vi "Final Project.vi"   [LabVIEW 2016, in "NEWNEW.lvrbt"]
uses:
  OneDrive/Documents/LabVIEW Data/NXTRobotics/Projects/NEWNEW/NEWNEW.lvrbt
  <vilib>/NXT/Block Support/NXT_InputPort.ctl
  <vilib>/NXT/Block Support/NXT_ButtonSelector.ctl
  <vilib>/NXT/Block Support/NXT_OutputPort.ctl
  <vilib>/NXT/Dual Mode Library/Sensors/EV3_Ultrasonic_CM.vi
  <vilib>/NXT/Dual Mode Library/Sensors/Light_On.vi
  <vilib>/NXT/NXTIO Xnodes/NXTIONodeSubVIs/NXTMoveMotors.vi
  <vilib>/NXT/NXTIO Xnodes/NXTIONodeSubVIs/NXTStopMotors.vi
  <vilib>/NXT/Subs/LVHSConnector.ctl
  <vilib>/NXT/NXTIO Xnodes/AddressXNode/NXTIOAddress.xnode
  <vilib>/NXT/NXTIO Xnodes/NXTIOXNode/NXTIO.xnode
  <vilib>/NXT/LegoClasses/BrickReference/BrickReference.lvclass
types:
  T1 = typedef "NXT_OutputPort.ctl" = u8
  T2 = typedef "NXT_ButtonSelector.ctl" = u16
  T3 = typedef "NXT_InputPort.ctl" = u32
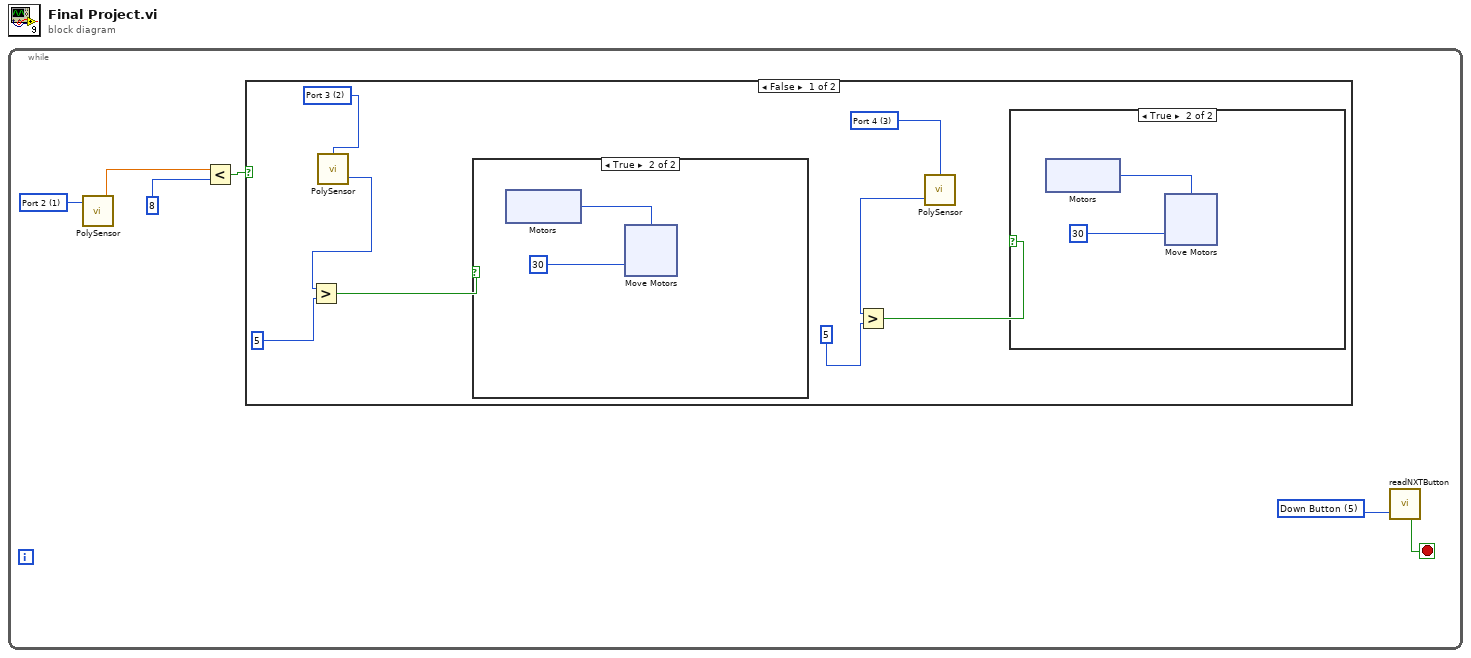
[diagram p0: block diagram]
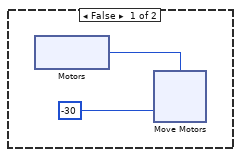
[diagram p2: hidden frame]
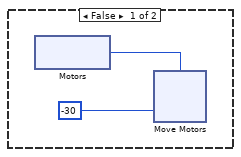
[diagram p3: hidden frame]
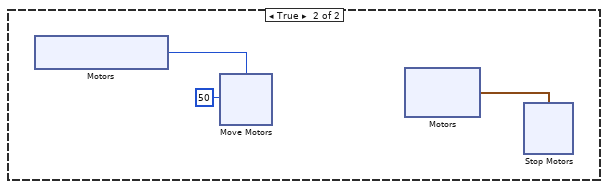
[diagram p4: hidden frame]
diagram:
  n1 = while {
    stop <- w1 stop-if-true
    w2 = T2 5 items=["Enter button"=3, "Left button"=2, "Right button"=1, "Up Button"=4, "Down Button"=5] ("Button (Enter button)")
    w6 = T3 1 items=["Port 1", "Port 2", "Port 3", "Port 4"] ("Port (Port 1)")
    n2 = call-poly <vilib>:"PolySensor.vi"("Port (Port 1)"=w6) -> ("Centimeters"=w4:sgl)  [unwired: 2 in, 1 out]
    n3 = Less?(x=w4, y=8) -> (x < y?=w3:bool)
    n4 = case shown="False" w3 {
      frame False {
        w7 = T3 3 items=["Port 1", "Port 2", "Port 3", "Port 4"] ("Port (Port 1)")
        w13 = T3 2 items=["Port 1", "Port 2", "Port 3", "Port 4"] ("Port (Port 1)")
        n5 = call-poly <vilib>:"PolySensor.vi"("Port (Port 3)"=w13) -> ("Scaled Value"=w14:i16)  [unwired: 2 in, 1 out]
        n6 = Greater?(x=w14, y=5) -> (0:w11:bool)
        n7 = case shown="True" w11 {
          frame False {
            n8 = xnode "Motors"() -> ("Motor"=w36:T1)
            n9 = xnode "Move Motors"("Power/Speed 1"=-30, "Motors"=w36) -> ()  [unwired: 1 in, 1 out]
          }
          frame True {
            n10 = xnode "Motors"() -> ("Motor"=w46:T1)
            n11 = xnode "Move Motors"("Power/Speed 1"=30, "Motors"=w46) -> ()  [unwired: 1 in, 1 out]
          }
        }
        n12 = call-poly <vilib>:"PolySensor.vi"("Port (Port 3)"=w7) -> ("Scaled Value"=w9:i16)  [unwired: 2 in, 1 out]
        n13 = Greater?(x=w9, y=5) -> (0:w8:bool)
        n14 = case shown="True" w8 {
          frame False {
            n15 = xnode "Motors"() -> ("Motor"=w16:T1)
            n16 = xnode "Move Motors"("Power/Speed 1"=-30, "Motors"=w16) -> ()  [unwired: 1 in, 1 out]
          }
          frame True {
            n17 = xnode "Motors"() -> ("Motor"=w26:T1)
            n18 = xnode "Move Motors"("Power/Speed 1"=30, "Motors"=w26) -> ()  [unwired: 1 in, 1 out]
          }
        }
      }
      frame True {
        n19 = xnode "Motors"() -> ("Motor"=w57:T1)
        n20 = xnode "Move Motors"("Power/Speed 1"=i8 50, "Motors"=w57) -> ()  [unwired: 1 in, 1 out]
        n21 = xnode "Motors"() -> ("Motor"=w55:cluster{"Port":T1, "Port":T1})
        n22 = xnode "Stop Motors"("Motors"=w55) -> ()  [unwired: 1 in, 1 out]
      }
    }
    n23 = call <vilib>:"readNXTButton.vi"("Button (Enter button)"=w2) -> ("Yes/No"=w1:bool)  [unwired: 2 in, 1 out]
  }
